vi "ep_Error Check (Multiple Lines).vi"(7 "reset? (F)":bool, 8 "error in (no error)":errorcluster, 9 "system info in":refnum<class "EP System Info.lvclass">, 11 "data in":sgl[][](array[numeric]) format="%#.21g") -> (0 "error out":errorcluster, 1 "system info out":refnum<class "EP System Info.lvclass">, 3 "data out":sgl[][](array[numeric]) format="%#.21g")   [LabVIEW 2014, in "NI_EP_Power Quality.lvlib"]
uses:
  <vilib>/addons/Electrical Power/PQ/NI_EP_Power Quality.lvlib
  <vilib>/addons/Electrical Power/PQ/Common/Classes/System Info/EP System Info.lvclass
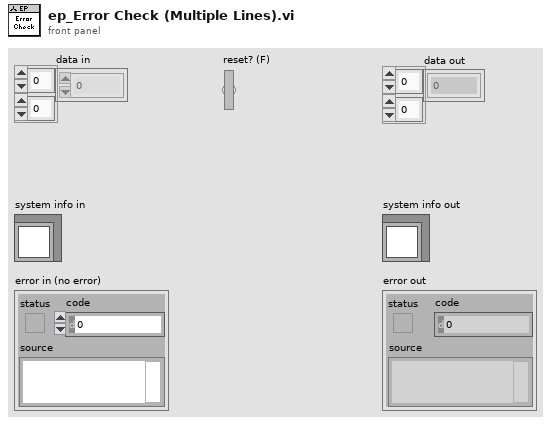
[diagram p1: front panel]
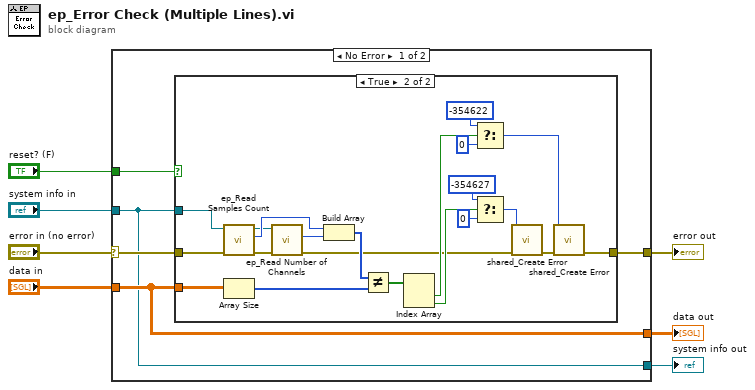
[diagram p0: block diagram]
diagram:
  n1 = case shown="No Error" "error in (no error)" {
    selector: "error in (no error)" -> [w12 w36]
    tunnel: "system info in" -> [w9 w35]
    tunnel: "data in" -> [w10 _]
    tunnel: [w11 w36] -> w4
    tunnel: [w10 _] -> w3
    tunnel: [w9 w35] -> w2
    tunnel: "reset? (F)" -> [w8 _]
    frame No Error {
      n2 = case shown="True" w8 {
        tunnel: w12 -> [w13 w34]
        tunnel: [w13 w33] -> w11
        tunnel: w10 -> [_ w32]
        tunnel: w9 -> [_ w31]
        frame False {
        }
        frame True {
          n3 = call <vilib>:"ep_Read Samples Count.vi"("error in (no error)"=w34, "system info in"=w31) -> ("error out"=w16:errorcluster, "basic calc. interval (samples)"=w18:i32, "system info out"=w17:refnum<class "EP System Info.lvclass">)  [unwired: 5 in, 2 out]
          n4 = Array Size(array=w32) -> (size(s)=w30:i32[])
          n5 = call <vilib>:"ep_Read Number of Channels.vi"("error in (no error)"=w16, "system info in"=w17) -> ("error out"=w15:errorcluster, "number of channels"=w14:i32)  [unwired: 7 in, 1 out]
          n6 = Build Array(w18, w14) -> (w29:i32[])
          n7 = Not Equal?(x=w29, y=w30) -> (x != y?=w25:bool[])
          n8 = Index Array(array=w25) -> (element #1=w24:bool, element #2=w23:bool)  [unwired: 2 in]
          n9 = Select(t=-354622, s=w24, f=0 ("error code (0)")) -> (s? t:f=w27:i32)
          n10 = Select(t=-354627, s=w23, f=0) -> (s? t:f=w19:i32)
          n11 = call <vilib>:"shared_Create Error.vi"("error in (no error)"=w15, "error code (0)"=w19) -> ("error out"=w20:errorcluster)  [unwired: 9 in]
          n12 = call <vilib>:"shared_Create Error.vi"("error in (no error)"=w20, "error code (0)"=w27) -> ("error out"=w33:errorcluster)  [unwired: 9 in]
        }
      }
    }
    frame Error {
    }
  }
  "error out" <- w4
  "data out" <- w3
  "system info out" <- w2
